vi "Calibration Rev1 (4).vi"() -> ()   [LabVIEW 2018]
uses:
  <vilib>/DAQmx/read.llb/DAQmx Read (Counter DBL 1Chan 1Samp).vi
  <vilib>/printing/EasyPrinting.llb/Easy Print VI Panel or Documentation (path).vi
  Counters.vi
  <vilib>/DAQmx/create/channels.llb/DAQmx Create Channel (CI-Frequency).vi
  <vilib>/DAQmx/miscellaneous.llb/DAQmx Fill In Error Info.vi
  <vilib>/Utility/NIReport.llb/NI_ReportGenerationCore.lvlib
  <vilib>/ptbypt/NI_PtbyPt.lvlib
panel:
  out "Sol Pwr Amps (0-2.5)":dbl format="%.3f"
  out "Sol Pwr Volts (Fixed 28)":dbl format="%.3f"
  out "TM2 Amps (0-.8)":dbl format="%.3f"
  out "TM2 Volts (0-35)":dbl format="%.3f"
  out "TM1 Amps (0-2)":dbl format="%.3f"
  out "Fuel RTD (EK-209)":dbl format="%.3f"
  out "Lube Temp Panel":dbl format="%.2f"
  out "Lube Res Temp":dbl format="%.2f"
  out "Fuel Temp (Panel)":dbl format="%.2f"
  out "Fuel Res Temp":dbl format="%.2f"
  out "TM1 Volts (0-35)":dbl format="%.3f"
  out "Fuel Level (0-2)":dbl format="%.3f"
  out "Lube Level (0-2)":dbl format="%.3f"
  out "Fuel DP3 (0-500)":dbl format="%.3f"
  out "Fuel DP2 (0-100)":dbl format="%.3f"
  out "Fuel DP1 (0-100)":dbl format="%.3f"
  out "Fuel P1 (0-1500)":dbl format="%.3f"
  out "Fuel P2 (0-1000)":dbl format="%.3f"
  out "Fuel P3 (0-1000)":dbl format="%.3f"
  out "Fuel P4 (0-1000)":dbl format="%.3f"
  out "Fuel P5 (0-600)":dbl format="%.3f"
  out "Fuel P6 (0-600)":dbl format="%.3f"
  out "Fuel P7 (0-200)":dbl format="%.3f"
  out "Fuel P8 (0-200)":dbl format="%.3f"
  out "Fuel P0 (0-200)":dbl format="%.3f"
  out "Lube P1 (0-50abs)":dbl format="%.3f"
  out "Lube P2 (0-50abs)":dbl format="%.3f"
  out "Lube P3 (0-600)":dbl format="%.3f"
  out "Lube P4 (0-200)":dbl format="%.3f"
  out "Lube P5 (0-200)":dbl format="%.3f"
  out "Lube P6 (0-200)":dbl format="%.3f"
  out "Lube P7 (0-200)":dbl format="%.3f"
  in  "st":bool
  in  "Print Screen":bool
  in  "Manual Zero":bool
  # "DAQ Calibration View"
  # "Lube"
  # "Fuel"
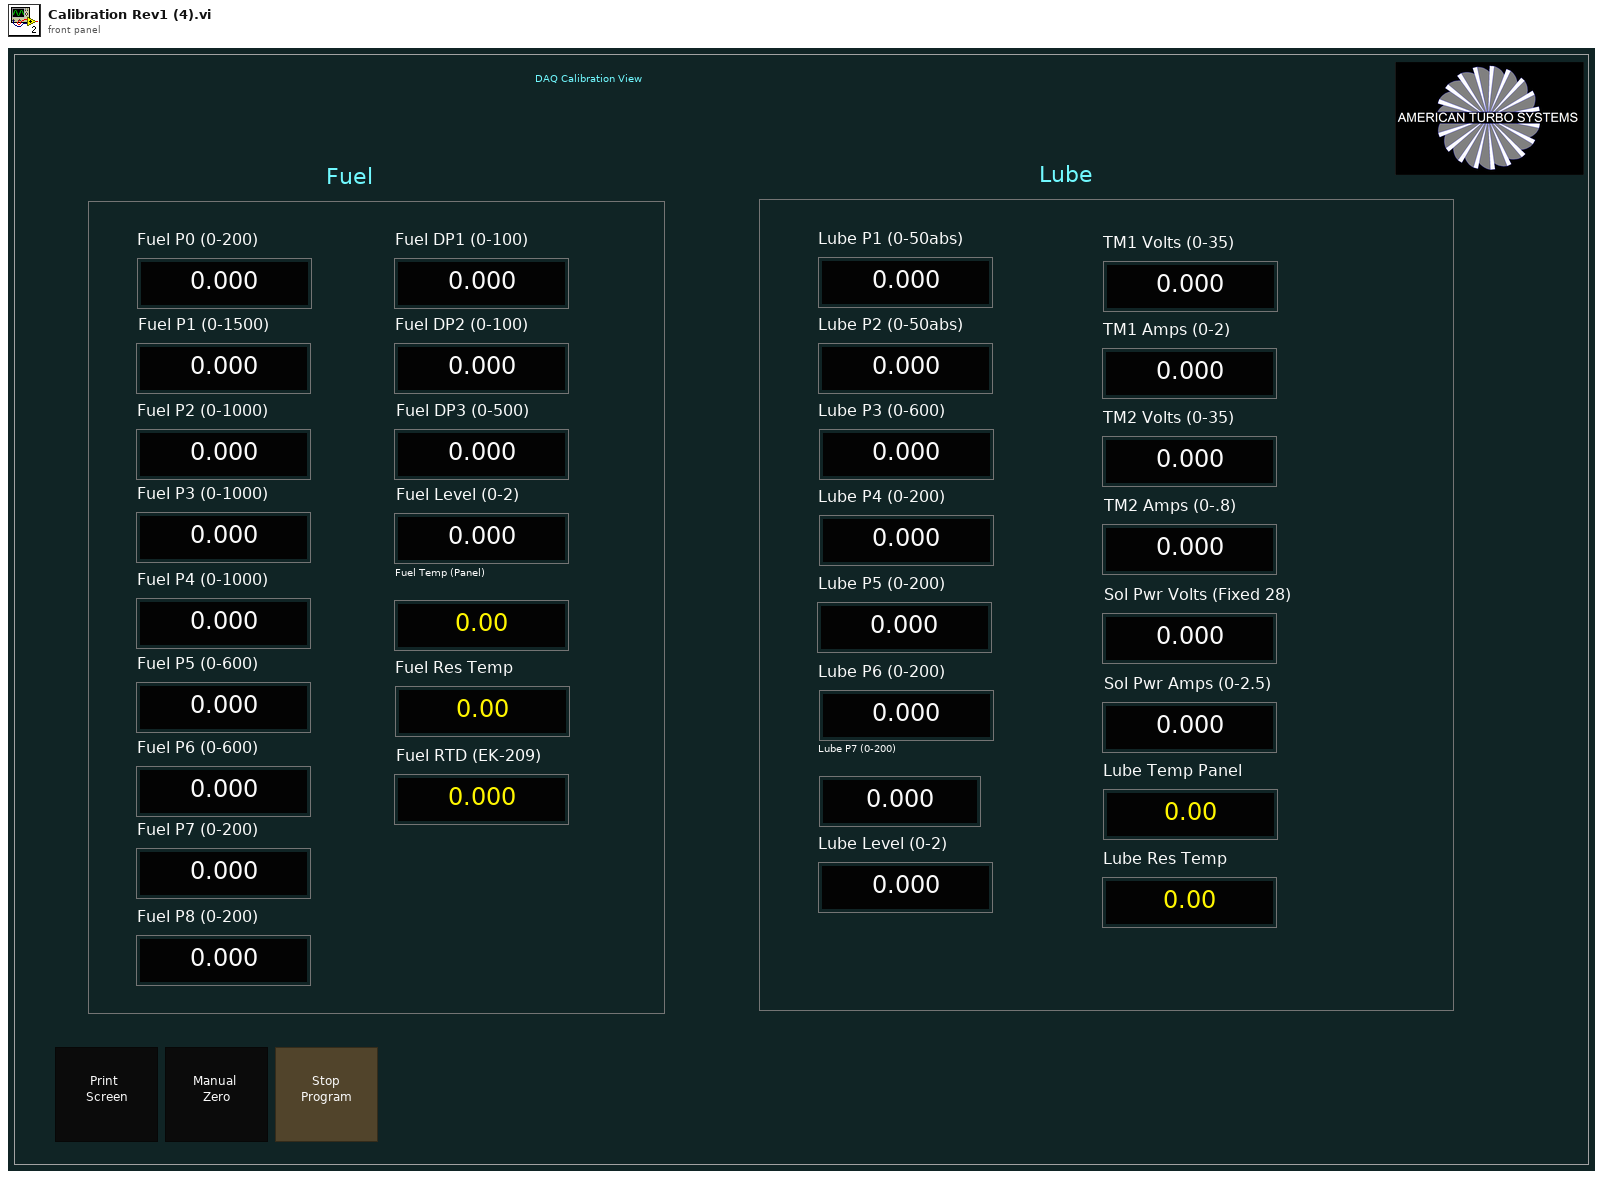
[diagram p1: front panel]
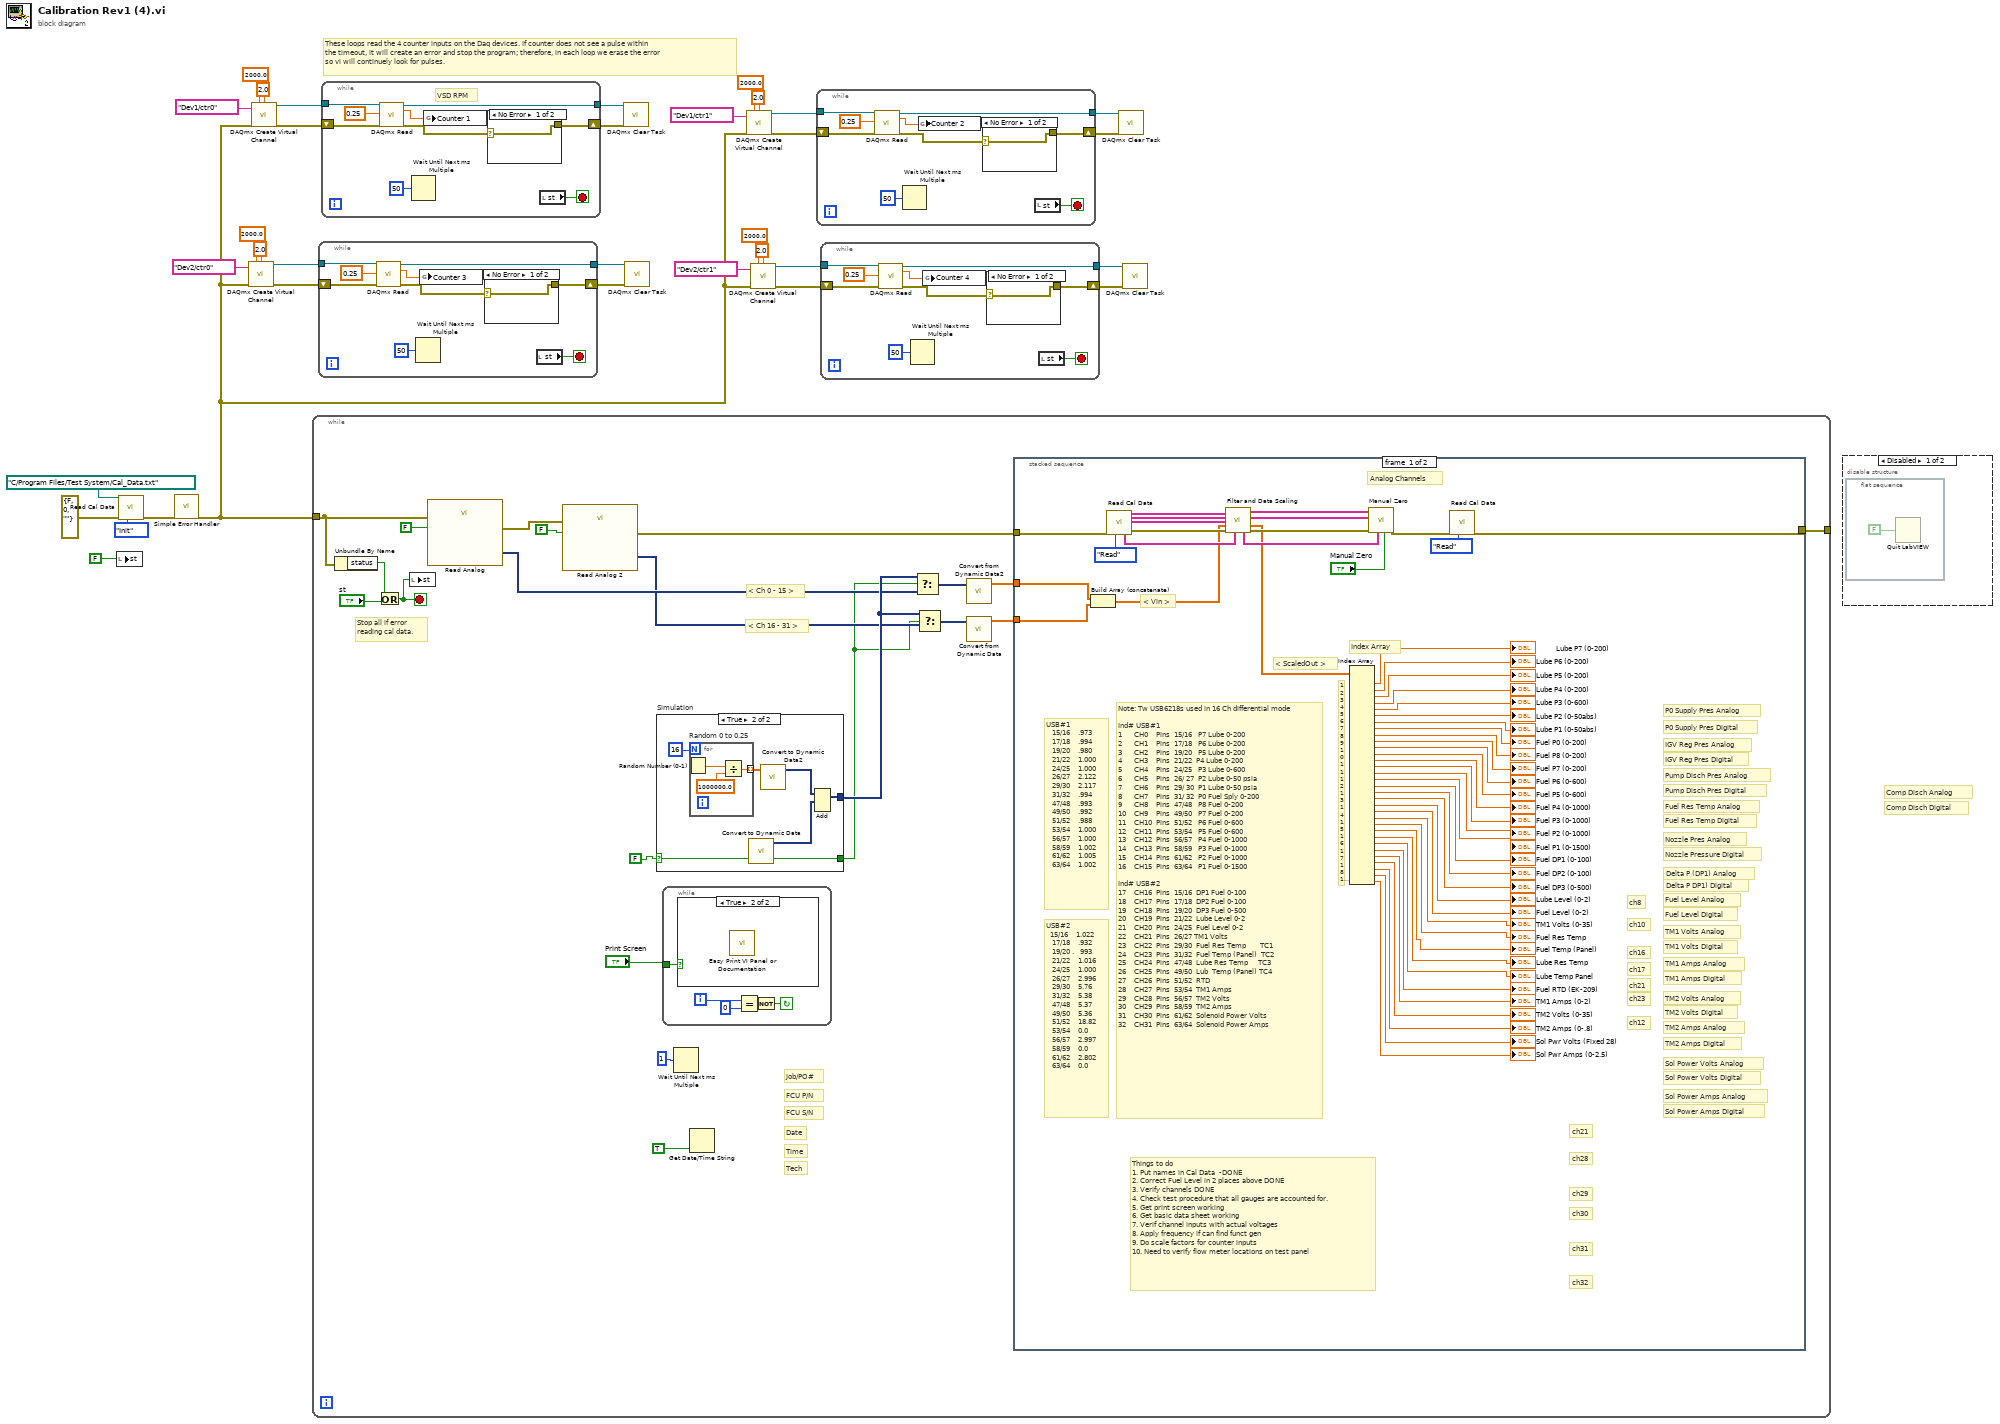
[diagram p0: block diagram]
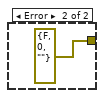
[diagram p2: hidden frame]
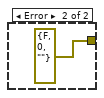
[diagram p3: hidden frame]
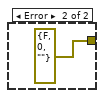
[diagram p4: hidden frame]
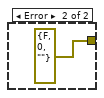
[diagram p5: hidden frame]
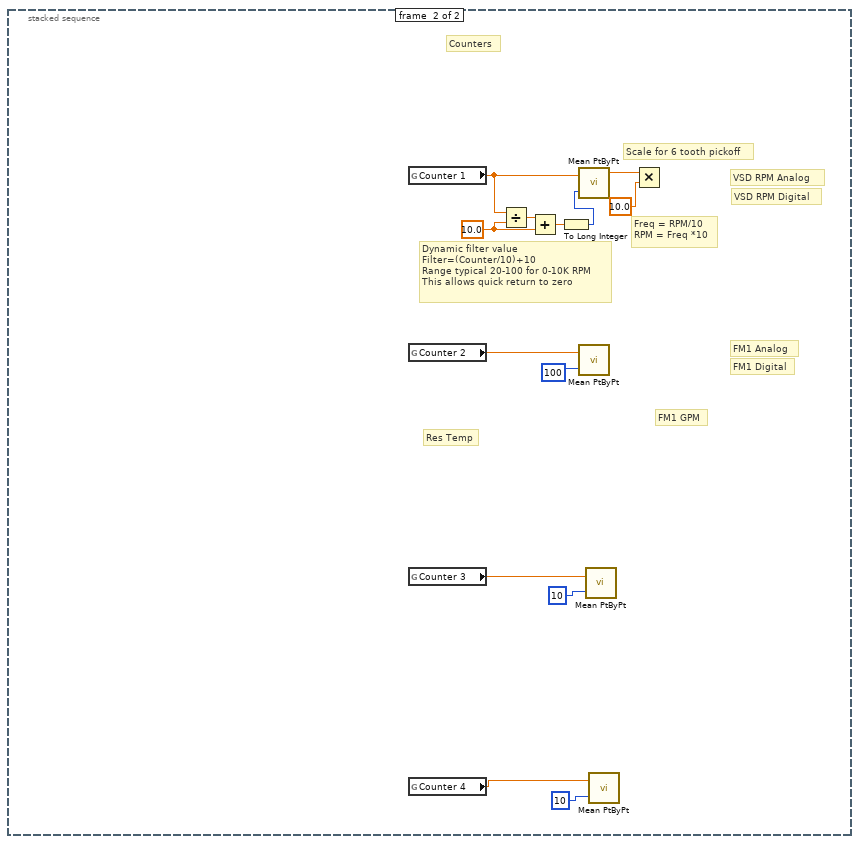
[diagram p9: hidden frame]
diagram:
  # "These loops read the 4 counter inputs on the Daq devices. If counter does not see a pulse within\nthe timeout, it will create an error and stop the program; therefore, in each loop we erase the error\nso vi will continuely look for pulses."
  # "Comp Disch Digital"
  # "Comp Disch Analog"
  n1 = local write "st"(FALSE ("stop")) -> ()
  n2 = call "Read Cal Data.vi"("Path"=path "C:/Program Files/Test System/Cal_Data.txt", "error in (no error)"=errorcluster {"status"=FALSE, "code"=0, "source"=""} ("error in"), "Enum"=enum16{"Init", "Read", "Write"}."Init") -> ("error out"=w32:errorcluster)  [unwired: 1 in, 11 out]
  n3 = call <vilib>:"Simple Error Handler.vi"("error in (no error)"=w32) -> ("error out"=w31:errorcluster)  [unwired: 1 in, 7 out]
  n4 = call-poly <vilib>:"DAQmx Create Virtual Channel.vi"("maximum value"=2000.0, "minimum value"=2.0, "counter"=tag "Dev2/ctr0", "error in"=w31) -> ("task out"=w29:refnum<k21>, "error out"=w24:errorcluster)  [unwired: 8 in, 2 out]
  n5 = call-poly <vilib>:"DAQmx Create Virtual Channel.vi"("maximum value"=2000.0, "minimum value"=2.0, "counter"=tag "Dev1/ctr0", "error in"=w31) -> ("task out"=w9:refnum<k21>, "error out"=w14:errorcluster)  [unwired: 8 in, 2 out]
  n6 = while {
    tunnel: w31 -> [w44]
    tunnel: [w45] -> _
    stop <- w42 stop-if-true
    # "Job/PO#"
    # "FCU P/N"
    # "FCU S/N"
    # "Date"
    # "Time"
    # "Tech"
    # "Stop all if error\nreading cal data."
    # "< Ch 16 - 31 >"
    # "< Ch 0 - 15 >"
    n7 = Unbundle By Name(w44) -> ("status"=w43:bool)
    n8 = Or(x=w43, y="st") -> (x .or. y?=w42:bool)
    n9 = local write "st"(w42) -> ()
    n10 = call "Read Analog"("error in"=w44, "stop (T)"=FALSE) -> ("data"=w50:dynamicdata, "error out"=w38:errorcluster)  [unwired: 1 in, 15 out]
    n11 = call "Read Analog 2"("error in"=w38, "stop (T)"=FALSE ("stop (F)")) -> ("data"=w49:dynamicdata, "error out"=w46:errorcluster)  [unwired: 1 in, 15 out]
    n12 = case "Simulation" shown="True" FALSE {
      selector: FALSE -> [w61 w62]
      tunnel: [_ w63] -> w52
      tunnel: [w61 w62] -> w48
      frame False {
        # "Using default if not wired-->"
        # "Do nothing"
      }
      frame True {
        n13 = for "Random 0 to 0.25" {
          N: 16 -> [_]
          tunnel: [w70] -> w67 mode=indexing
          n14 = Random Number (0-1)() -> (number: 0 to 1=w69:dbl)
          n15 = Divide(x=w69, y=1000000.0) -> (x/y=w70:dbl)
        }
        n16 = call "Convert to Dynamic Data"() -> ("Dynamic Data Type"=w65:dynamicdata)  [unwired: 1 in, 3 out]
        n17 = call "Convert to Dynamic Data2"("Array"=w67) -> ("Dynamic Data Type"=w64:dynamicdata)  [unwired: 3 out]
        n18 = Add(1:w65, 2:w64) -> (0:w63:dynamicdata)  [unwired: 1 in, 1 out]
      }
    }
    n19 = while {
      tunnel: "Print Screen" -> [w60]
      i -> [w58]
      stop <- w56 continue-if-true
      n20 = case shown="True" w60 {
        frame False {
          # "Do nothing"
        }
        frame True {
          n21 = call-poly <vilib>:"Easy Print VI Panel or Documentation.vi"() -> ()  [unwired: 4 in, 8 out]
        }
      }
      n22 = Equal?(x=w58, y=0) -> (x = y?=w57:bool)
      n23 = Not(x=w57) -> (.not. x?=w56:bool)
    }
    n24 = Wait Until Next ms Multiple(millisecond multiple=u32 1) -> ()  [unwired: 1 out]
    n25 = Get Date/Time String(want seconds? (F)=TRUE) -> ()  [unwired: 4 out]
    n26 = Select(t=w52, s=w48, f=w50) -> (s? t:f=w53:dynamicdata)
    n27 = Select(t=w52, s=w48, f=w49) -> (s? t:f=w55:dynamicdata)
    n28 = call "Convert from Dynamic Data2"("Dynamic Data Type"=w53) -> ("Array"=w51:dbl[])  [unwired: 3 out]
    n29 = call "Convert from Dynamic Data"("Dynamic Data Type"=w55) -> ("Array"=w54:dbl[])  [unwired: 3 out]
    n30 = stacked-sequence {
      tunnel: w54 -> [w110 _]
      tunnel: w51 -> [w109 _]
      tunnel: w46 -> [w121 _]
      tunnel: [w106 _] -> w45
      frame #0 {
        # "ch21"
        # "ch17"
        # "Delta P DP1) Digital"
        # "Delta P (DP1) Analog"
        # "ch10"
        # "IGV Reg Pres Digital"
        # "IGV Reg Pres Analog"
        # "USB#2\t\n  15/16\t   1.022\n   17/18\t   .932\n   19/20\t.   993\n   21/22\t   1.016\n   24/25\t   1.000\n   26/27\t   2.996\n   29/30\t   5.76\n   31/32\t   5.38\n   47/48\t   5.37\n   49/50\t   5.36\n   51/52\t   18.82\n   53/54\t   0.0\n   56/57\t   2.997\n   58/59\t   0.0\n   61/62\t   2.802\n   63/64\t   0.0"
        # "Things to do\n1. Put names in Cal Data  -DONE\n2. Correct Fuel Level in 2 places above DONE\n3. Verify channels DONE\n4. Check test procedure that all gauges are accounted for.\n5. Get print screen working\n6. Get basic data sheet working\n7. Verif channel inputs with actual voltages\n8. Apply frequency if can find funct gen\n9. Do scale factors for counter inputs\n10. Need to verify flow meter locations on test panel"
        # "ch12"
        # "Nozzle Pressure Digital"
        # "Nozzle Pres Analog"
        # "ch21"
        # "ch32"
        # "ch31"
        # "ch30"
        # "ch29"
        # "TM1 Amps Digital"
        # "TM1 Amps Analog"
        # "TM1 Volts Digital"
        # "TM1 Volts Analog"
        # "TM2 Amps Digital"
        # "TM2 Amps Analog"
        # "TM2 Volts Digital"
        # "TM2 Volts Analog"
        # "Sol Power Amps Digital"
        # "Sol Power Amps Analog"
        # "Sol Power Volts Digital"
        # "Sol Power Volts Analog"
        # "ch16"
        # "ch23"
        # "Fuel Res Temp Analog"
        # "Fuel Res Temp Digital"
        # "USB#1\t\n   15/16   \t.973\n   17/18\t   .994\n   19/20\t   .980\n   21/22\t   1.000\n   24/25\t   1.000\n   26/27\t   2.122\n   29/30\t   2.117\n   31/32\t   .994\n   47/48\t   .993\n   49/50\t   .992\n   51/52\t   .988\n   53/54\t   1.000\n   56/57\t   1.000\n   58/59\t   1.002\n   61/62\t   1.005\n   63/64\t   1.002"
        # "1\n2\n3\n4\n5\n6\n7\n8\n9\n10\n11\n12\n13\n14\n15\n16\n17\n18\n19\n20\n21\n22\n23\n24\n25\n26\n27\n28\n29\n30\n31\n32"
        # "Fuel Level Analog"
        # "Fuel Level Digital"
        # "ch28"
        # "Pump Disch Pres Digital"
        # "Pump Disch Pres Analog"
        # "ch8"
        # "Index Array"
        # "P0 Supply Pres Digital"
        # "P0 Supply Pres Analog"
        # "< ScaledOut >"
        # "< Vin >"
        # "Note: Tw USB6218s used in 16 Ch differential mode\n\nInd# USB#1\n1      CH0\t\t  Pins  15/16\t  P7 Lube 0-200\n2      CH1\t\t  Pins  17/18\t  P6 Lube 0-200\n3      CH2\t\t  Pins  19/20   P5 Lube 0-200\n4      CH3\t\t  Pins  21/22  P4 Lube 0-200\n5      CH4\t   Pins  24/25\t  P3 Lube 0-600\n6      CH5\t\t  Pins  26/\t27\t P2 Lube 0-50 psia\n7      CH6\t   Pins  29/\t30\t P1 Lube 0-50 psia\n8      CH7\t  \tPins  31/ 32\t P0 Fuel Sply 0-200  \n9      CH8\t  \tPins  47/48\t  P8 Fuel 0-200   \n10    CH9\t\t  Pins  49/50\t  P7 Fuel 0-200   \n11    CH10\t\tPins  51/52\t  P6 Fuel 0-600   \n12    CH11\t\tPins  53/54\t  P5 Fuel 0-600   \n13    CH12\t\tPins  56/57\t  P4 Fuel 0-1000 \n14    CH13\t\tPins  58/59\t  P3 Fuel 0-1000 \n15    CH14\t\tPins  61/62 \t P2 Fuel 0-1000  \n16    CH15\t\tPins  63/64 \t P1 Fuel 0-1500 \n\nInd# USB#2\n17    CH16\t\tPins  15/16\t DP1 Fuel 0-100 \n18    CH17\t\tPins  17/18\t DP2 Fuel 0-100\n19    CH18\t\tPins  19/20  DP3 Fuel 0-500 \n20    CH19\t Pins  21/22\t Lube Level 0-2 \n21    CH20\t\tPins  24/25\t Fuel Level 0-2 \n22    CH21\t\tPins  26/27\tTM1 Volts  \n23    CH22\t Pins  29/30  Fuel Res Temp       TC1\n24    CH23\t\tPins  31/32\t Fuel Temp (Panel)  TC2 \n25    CH24\t\tPins \t47/48\t Lube Res Temp     TC3 \n26    CH25\t\tPins  49/50\t Lub  Temp (Panel) TC4 \n27    CH26\t\tPins  51/52\t RTD \n28    CH27\t\tPins  53/54\t TM1 Amps \n29    CH28\t\tPins  56/57\t TM2 Volts\n30    CH29\t\tPins  58/59\t TM2 Amps \n31    CH30\t\tPins  61/62  Solenoid Power Volts \n32    CH31\t\tPins  63/64  Solenoid Power Amps"
        # "Analog Channels"
        n31 = Build Array (concatenate)(w109, w110) -> (w104:dbl[])
        n32 = call "Read Cal Data.vi"("error in (no error)"=w121, "Enum"=enum16{"Init", "Read", "Write"}."Read") -> ("Offset"=w119:string[], "Slope"=w118:string[], "Filter"=w117:string[], "Allow Zero?"=w120:string[], "error out"=w115:errorcluster)  [unwired: 2 in, 7 out]
        n33 = call "Filter and Data Scaling.vi"("Offset Data"=w119, "Slope Data"=w118, "Filter Data"=w117, "Vin"=w104, "error in"=w115, "Allow Zero?"=w120) -> ("Vout"=w111:string[], "Offset Data"=w112:string[], "ScaledOut"=w103:dbl[], "Allow Zero?"=w116:string[], "error out"=w114:errorcluster)  [unwired: 5 out]
        n34 = Index Array(array=w103) -> (element #1=→"Lube P7 (0-200)":dbl, element #2=→"Lube P6 (0-200)":dbl, element #3=→"Lube P5 (0-200)":dbl, element #4=→"Lube P4 (0-200)":dbl, element #5=→"Lube P3 (0-600)":dbl, element #6=→"Lube P2 (0-50abs)":dbl, element #7=→"Lube P1 (0-50abs)":dbl, element #8=→"Fuel P0 (0-200)":dbl, element #9=→"Fuel P8 (0-200)":dbl, element #10=→"Fuel P7 (0-200)":dbl, element #11=→"Fuel P6 (0-600)":dbl, element #12=→"Fuel P5 (0-600)":dbl, element #13=→"Fuel P4 (0-1000)":dbl, element #14=→"Fuel P3 (0-1000)":dbl, element #15=→"Fuel P2 (0-1000)":dbl, element #16=→"Fuel P1 (0-1500)":dbl, element #17=→"Fuel DP1 (0-100)":dbl, element #18=→"Fuel DP2 (0-100)":dbl, element #19=→"Fuel DP3 (0-500)":dbl, element #20=→"Lube Level (0-2)":dbl, element #21=→"Fuel Level (0-2)":dbl, element #22=→"TM1 Volts (0-35)":dbl, element #23=→"Fuel Res Temp":dbl, element #24=→"Fuel Temp (Panel)":dbl, element #25=→"Lube Res Temp":dbl, element #26=→"Lube Temp Panel":dbl, element #27=→"Fuel RTD (EK-209)":dbl, element #28=→"TM1 Amps (0-2)":dbl, element #29=→"TM2 Volts (0-35)":dbl, element #30=→"TM2 Amps (0-.8)":dbl, element #31=→"Sol Pwr Volts (Fixed 28)":dbl, element #32=→"Sol Pwr Amps (0-2.5)":dbl)  [unwired: 32 in]
        n35 = call "Manual Zero.vi"("Manual Zero"="Manual Zero", "Allow Zero?"=w116, "error in"=w114, "Offset Data"=w112, "Vin"=w111) -> ("error out"=w107:errorcluster)  [unwired: 6 out]
        n36 = call "Read Cal Data.vi"("error in (no error)"=w107, "Enum"=enum16{"Init", "Read", "Write"}."Read") -> ("error out"=w106:errorcluster)  [unwired: 2 in, 11 out]
      }
      frame #1 {
        w123 = 10.0
        # "Dynamic filter value\nFilter=(Counter/10)+10\nRange typical 20-100 for 0-10K RPM\nThis allows quick return to zero"
        # "Freq = RPM/10\nRPM = Freq *10"
        # "Scale for 6 tooth pickoff"
        # "Res Temp"
        # "FM1 GPM"
        # "FM1 Digital"
        # "FM1 Analog"
        # "VSD RPM Digital"
        # "VSD RPM Analog"
        # "Counters"
        n37 = global read "Counters.vi" "Counter 1"() -> (w126:dbl)
        n38 = global read "Counters.vi" "Counter 2"() -> (w133:dbl)
        n39 = global read "Counters.vi" "Counter 3"() -> (w131:dbl)
        n40 = global read "Counters.vi" "Counter 4"() -> (w129:dbl)
        n41 = Divide(x=w126, y=w123) -> (x/y=w124:dbl)
        n42 = Add(x=w124, y=w123) -> (x+y=w122:dbl)
        n43 = To Long Integer(number=w122) -> (32bit integer=w125:i32)
        n44 = call <vilib>:"Mean PtByPt.vi"("x"=w126, "sample length"=w125) -> ("mean"=w128:dbl)  [unwired: 1 in, 2 out]
        n45 = call <vilib>:"Mean PtByPt.vi"("x"=w133, "sample length"=100) -> ()  [unwired: 1 in, 3 out]
        n46 = call <vilib>:"Mean PtByPt.vi"("x"=w131, "sample length"=10) -> ()  [unwired: 1 in, 3 out]
        n47 = call <vilib>:"Mean PtByPt.vi"("x"=w129, "sample length"=10) -> ()  [unwired: 1 in, 3 out]
        n48 = Multiply(x=w128, y=10.0) -> ()  [unwired: 1 out]
      }
    }
  }
  n49 = while {
    tunnel: w29 -> [w143]
    tunnel: [w142] -> w25
    shift-right: [w138] -> w23
    shift-left: w24 -> [w140]
    stop <- w141 stop-if-true
    n50 = call-poly <vilib>:"DAQmx Read.vi"("task/channels in"=w143, "timeout"=0.25, "error in"=w140) -> ("task out"=w142:refnum<k21>, "data"=w136:dbl, "error out"=w139:errorcluster)  [unwired: 10 out]
    n51 = Wait Until Next ms Multiple(millisecond multiple=u32 50) -> ()  [unwired: 1 out]
    n52 = global write "Counters.vi" "Counter 3"(w136) -> ()
    n53 = case shown="No Error" w139 {
      selector: w139 -> [w144 _]
      tunnel: [w144 errorcluster {"status"=FALSE, "code"=0, "source"=""} ("error IO")] -> w138
      frame No Error {
      }
      frame Error {
      }
    }
    n54 = local read "st"() -> (w141:bool)
  }
  n55 = while {
    tunnel: w9 -> [w154]
    tunnel: [w153] -> w13
    shift-right: [w149] -> w15
    shift-left: w14 -> [w151]
    stop <- w152 stop-if-true
    # "VSD RPM"
    n56 = call-poly <vilib>:"DAQmx Read.vi"("task/channels in"=w154, "timeout"=0.25, "error in"=w151) -> ("task out"=w153:refnum<k21>, "data"=w147:dbl, "error out"=w150:errorcluster)  [unwired: 10 out]
    n57 = Wait Until Next ms Multiple(millisecond multiple=u32 50) -> ()  [unwired: 1 out]
    n58 = global write "Counters.vi" "Counter 1"(w147) -> ()
    n59 = case shown="No Error" w150 {
      selector: w150 -> [w155 _]
      tunnel: [w155 errorcluster {"status"=FALSE, "code"=0, "source"=""} ("error IO")] -> w149
      frame No Error {
      }
      frame Error {
      }
    }
    n60 = local read "st"() -> (w152:bool)
  }
  n61 = call <vilib>:"DAQmx Clear Task.vi"("task in"=w13, "error in"=w15) -> ()  [unwired: 14 out]
  n62 = call <vilib>:"DAQmx Clear Task.vi"("task in"=w25, "error in"=w23) -> ()  [unwired: 14 out]
  n63 = call-poly <vilib>:"DAQmx Create Virtual Channel.vi"("maximum value"=2000.0, "minimum value"=2.0, "counter"=tag "Dev1/ctr1", "error in"=w31) -> ("task out"=w8:refnum<k21>, "error out"=w3:errorcluster)  [unwired: 8 in, 2 out]
  n64 = call-poly <vilib>:"DAQmx Create Virtual Channel.vi"("maximum value"=2000.0, "minimum value"=2.0, "counter"=tag "Dev2/ctr1", "error in"=w31) -> ("task out"=w16:refnum<k21>, "error out"=w21:errorcluster)  [unwired: 8 in, 2 out]
  n65 = while {
    tunnel: w8 -> [w165]
    tunnel: [w164] -> w4
    shift-right: [w160] -> w2
    shift-left: w3 -> [w162]
    stop <- w163 stop-if-true
    n66 = call-poly <vilib>:"DAQmx Read.vi"("task/channels in"=w165, "timeout"=0.25, "error in"=w162) -> ("task out"=w164:refnum<k21>, "data"=w158:dbl, "error out"=w161:errorcluster)  [unwired: 10 out]
    n67 = Wait Until Next ms Multiple(millisecond multiple=u32 50) -> ()  [unwired: 1 out]
    n68 = global write "Counters.vi" "Counter 2"(w158) -> ()
    n69 = case shown="No Error" w161 {
      selector: w161 -> [w166 _]
      tunnel: [w166 errorcluster {"status"=FALSE, "code"=0, "source"=""} ("error IO")] -> w160
      frame No Error {
      }
      frame Error {
      }
    }
    n70 = local read "st"() -> (w163:bool)
  }
  n71 = while {
    tunnel: w16 -> [w176]
    tunnel: [w175] -> w20
    shift-right: [w171] -> w22
    shift-left: w21 -> [w173]
    stop <- w174 stop-if-true
    n72 = call-poly <vilib>:"DAQmx Read.vi"("task/channels in"=w176, "timeout"=0.25, "error in"=w173) -> ("task out"=w175:refnum<k21>, "data"=w169:dbl, "error out"=w172:errorcluster)  [unwired: 10 out]
    n73 = Wait Until Next ms Multiple(millisecond multiple=u32 50) -> ()  [unwired: 1 out]
    n74 = global write "Counters.vi" "Counter 4"(w169) -> ()
    n75 = case shown="No Error" w172 {
      selector: w172 -> [w177 _]
      tunnel: [w177 errorcluster {"status"=FALSE, "code"=0, "source"=""} ("error IO")] -> w171
      frame No Error {
      }
      frame Error {
      }
    }
    n76 = local read "st"() -> (w174:bool)
  }
  n77 = call <vilib>:"DAQmx Clear Task.vi"("task in"=w4, "error in"=w2) -> ()  [unwired: 14 out]
  n78 = call <vilib>:"DAQmx Clear Task.vi"("task in"=w20, "error in"=w22) -> ()  [unwired: 14 out]
  n79 = disable-structure shown="Disabled" {
    frame Disabled {
      n80 = flat-sequence {
        frame #0 {
          n81 = Quit LabVIEW(quit? (T)=FALSE) -> ()
        }
      }
    }
    frame Enabled {
    }
  }
